vi "Run.vi"(8 "error in (no error)":errorcluster, 11 "LV Server in":refnum<class "LV Server.lvclass">) -> (0 "error out":errorcluster, 3 "LV Server out":refnum<class "LV Server.lvclass">)   [LabVIEW 2020, in "LV Server.lvclass"]
uses:
  LV Server.lvclass
  LV Server.lvclass/LV Server.ctl
  f458beeb-ec7d-4c6f-b459-d8ae3f520d1c.vi
  Common/Message ID.ctl
  Common/Common.lvlib
  07a9a727-0d85-41e2-946b-274d381dcb4a.vi
panel:
  out "URL":string
  out "State":string
  out "Value":string
  in  "Reset":bool
  in  "Pause":bool
  in  "Start":bool
  # "Close the window to stop the server."
  # "Navigate a browser to the following URL to run a browser client:"
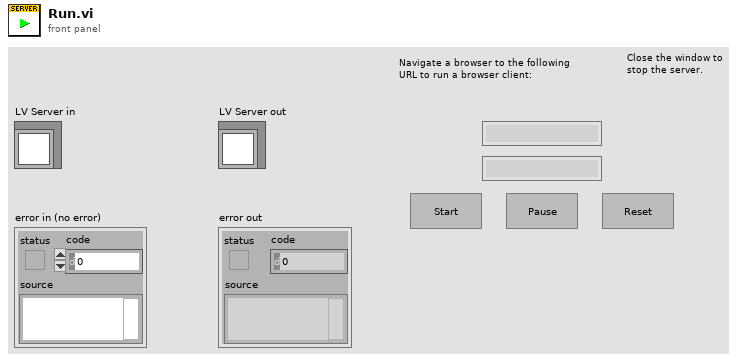
[diagram p1: front panel]
types:
  T1 = typedef "Common.lvlib/Message ID.ctl" = enum16{"Timer State", "Timer Value", "Timer Start", "Timer Pause", "Timer Reset", "Timer Init"}
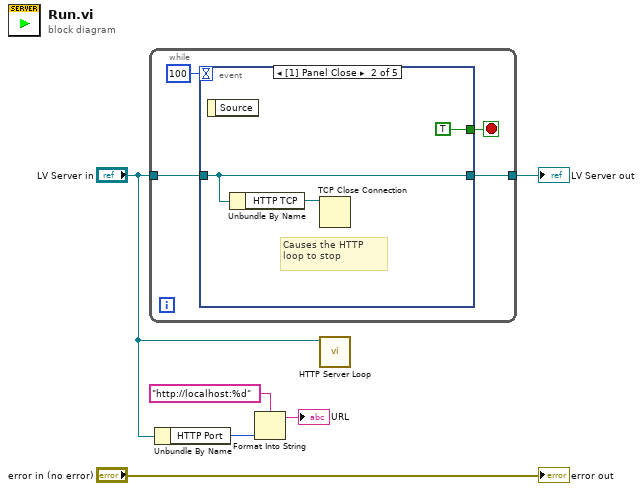
[diagram p0: block diagram]
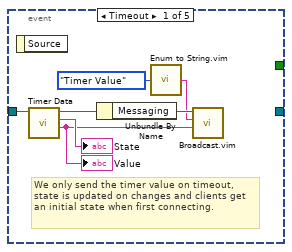
[diagram p2: hidden frame]
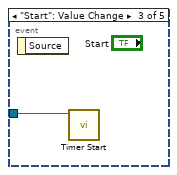
[diagram p3: hidden frame]
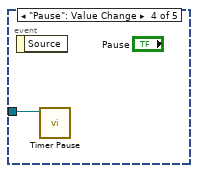
[diagram p4: hidden frame]
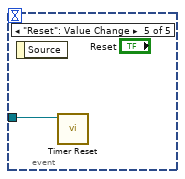
[diagram p5: hidden frame]
diagram:
  n1 = while {
    tunnel: "LV Server in" -> [w10]
    tunnel: [w7] -> w5
    stop <- w8 stop-if-true
    n2 = event shown="[1] Panel Close" {
      selector: _ -> [_ _ _ _ _]
      dyn-events: _ -> [_ _ _ _ _]
      timeout: 100 -> [_ _ _ _ _]
      tunnel: w10 -> [w17 w19 w21 w22 w23]
      tunnel: [_ TRUE _ _ _] -> w8
      tunnel: [_ w19 _ _ _] -> w7
      event Timeout {
        # "We only send the timer value on timeout, state is updated on changes and clients get an initial state when first connecting."
        n3 = event-data() -> ()  [unwired: 1 in, 1 out]
        n4 = call "Timer Data.vi"("LV Server in"=w17) -> ("Timer Value"=w13:string, "Timer State"=→"State":string, "LV Server out"=w15:refnum<class "LV Server.lvclass">)  [unwired: 7 in, 1 out]
        "Value" <- w13
        n5 = Unbundle By Name(w15) -> ("Messaging"=w14:refnum<class "Manager.lvclass">)
        n6 = call "Enum to String.vim"("Enum"=Message_ID."Timer Value" ("Message ID")) -> ("Enum String"=w11:string)
        n7 = call "Broadcast.vim"("Data"=w13, "ID"=w11, "Manager in"=w14) -> ()  [unwired: 7 in, 2 out]
      }
      event Panel Close {
        # "Causes the HTTP loop to stop"
        n8 = event-data() -> ()  [unwired: 1 in, 1 out]
        n9 = Unbundle By Name(w19) -> ("HTTP TCP"=w18:refnum<k5>)
        n10 = TCP Close Connection(connection ID=w18) -> ()  [unwired: 2 in, 2 out]
      }
      event "Start": Value Change {
        n11 = event-data() -> ()  [unwired: 1 in, 1 out]
        n12 = call "Timer Start.vi"("LV Server in"=w21) -> ()  [unwired: 9 in, 2 out]
      }
      event "Pause": Value Change {
        n13 = event-data() -> ()  [unwired: 1 in, 1 out]
        n14 = call "Timer Pause.vi"("LV Server in"=w22) -> ()  [unwired: 9 in, 2 out]
      }
      event "Reset": Value Change {
        n15 = event-data() -> ()  [unwired: 1 in, 1 out]
        n16 = call "Timer Reset.vi"("LV Server in"=w23) -> ()  [unwired: 9 in, 2 out]
      }
    }
  }
  "LV Server out" <- w5
  n17 = Unbundle By Name("LV Server in") -> ("HTTP Port"=w2:u16)
  n18 = Format Into String(format string="http://localhost:%d", w2) -> (resulting string=→"URL":string)  [unwired: 2 in, 1 out]
  n19 = call "HTTP Server Loop.vi"("LV Server in"="LV Server in") -> ()  [unwired: 10 in, 1 out]
  "error out" <- "error in (no error)"
